vi "create_channels_AO.vi"(0 "task in":refnum<k21>, 11 "error in":errorcluster) -> (4 "task out":refnum<k21>, 15 "error out":errorcluster)   [LabVIEW 2016]
uses:
  <vilib>/DAQmx/create/scale.llb/DAQmx Create Scale (Linear).vi
  <vilib>/DAQmx/create/channels.llb/DAQmx Create Channel (AO-Voltage-Basic).vi
panel:
  in  "y-intercept":dbl[](array[numeric])=[32.0, 32.0, 32.0, 32.0]
  in  "slope":dbl[](array[numeric])=[4.0, 4.0, 4.0, 4.0]
  in  "maximum":dbl[](array[numeric])=[52.0, 52.0, 52.0, 52.0]
  in  "minimum":dbl[](array[numeric])=[12.0, 12.0, 12.0, 12.0]
  in  "output terminal configuration":i32[](array[ring])=[10083, 10083, 10083, 10083] items=["default"=-1, "RSE"=10083, "NRSE"=10078, "Differential"=10106, "Pseudodifferential"=12529]
  in  "AO Temperature":tag[](array[tag])=["Dev1/ao1", "Dev1/ao0", "Dev1/ao3", "Dev1/ao2"]
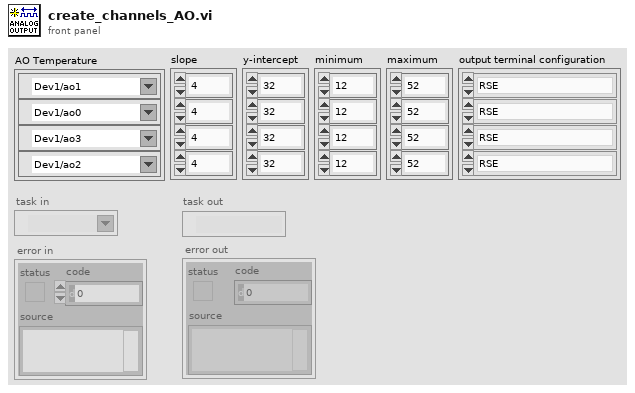
[diagram p1: front panel]
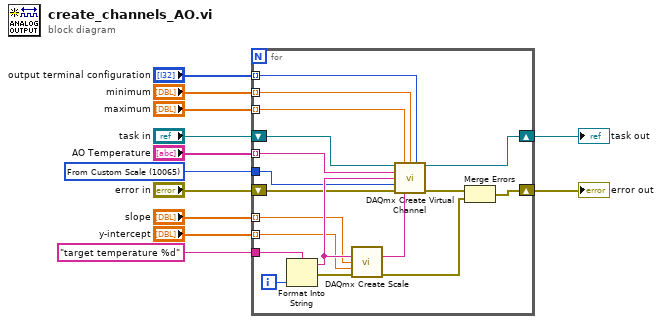
[diagram p0: block diagram]
diagram:
  w6 = 10065 items=["Volts"=10348, "From Custom Scale"=10065] ("units")
  n1 = for {
    tunnel: "AO Temperature" -> [w29] mode=indexing
    tunnel: "target temperature %d" ("name") -> [w28]
    tunnel: "y-intercept" -> [w24] mode=indexing
    tunnel: "slope" -> [w23] mode=indexing
    tunnel: w6 -> [w20]
    shift-right: [w15] -> w1
    shift-left: "error in" -> [w21]
    shift-right: [w19] -> w2
    shift-left: "task in" -> [w30]
    tunnel: "maximum" -> [w18] mode=indexing
    tunnel: "minimum" -> [w17] mode=indexing
    tunnel: "output terminal configuration" -> [w16] mode=indexing
    i -> [w27]
    n2 = Format Into String(format string=w28, w27) -> (resulting string=w25:string, error out=w26:errorcluster)  [unwired: 2 in]
    n3 = call-poly <vilib>:"DAQmx Create Scale.vi"("name"=w25, "slope"=w23, "y-intercept"=w24, "error in"=w26) -> ("scale out"=w22:tag, "error out"=w13:errorcluster)  [unwired: 10 in]
    n4 = call-poly <vilib>:"DAQmx Create Virtual Channel.vi"("task in"=w30, "maximum value"=w18, "minimum value"=w17, "output terminal configuration"=w16, "physical channels"=w29, "name to assign"=w25, "units"=w20, "error in"=w21, "custom scale name"=w22) -> ("task out"=w19:refnum<k21>, "error out"=w14:errorcluster)  [unwired: 5 in]
    n5 = Merge Errors(w14, w13) -> (w15:errorcluster)
  }
  "task out" <- w2
  "error out" <- w1
